vi "FPGA Read FIFO By Name - U32.vi"(6 "Timeout (ms)":u32=5000, 8 "error in (no error)":errorcluster, 9 "Number of Elements":u32, 10 "FIFO":string, 11 "FPGA Session In":refnum<class "FPGA Interface Base.lvclass">) -> (0 "error out":errorcluster, 1 "Elements Remaining":u32, 2 "Data":u32[](array[numeric]), 3 "FPGA Session Out":refnum<class "FPGA Interface Base.lvclass">)   [LabVIEW 2010, in "FPGA Interface Base.lvclass"]
doc: "Reads from a FIFO of unsigned 32-bit integers."
uses:
  <userlib>/_FPGA Interface Advanced Tools/FPGA Interface Base/FPGA Interface Base.lvclass
  <vilib>/rvi/DataTransferAndStorage/Container/Common/niFpgaDataTypeControl.ctl
  <userlib>/_FPGA Interface Advanced Tools/FPGA Interface Base/FPGA Interface Base.lvclass/FPGA Interface Base.ctl
  <vilib>/Utility/error.llb/Error Cluster From Error Code.vi
  <userlib>/_FPGA Interface Advanced Tools/FPGA Interface Base/Accessors/FPGA Read Session.vi
  <userlib>/_FPGA Interface Advanced Tools/FPGA Interface Wrapper/FPGA Interface Wrapper.lvlib
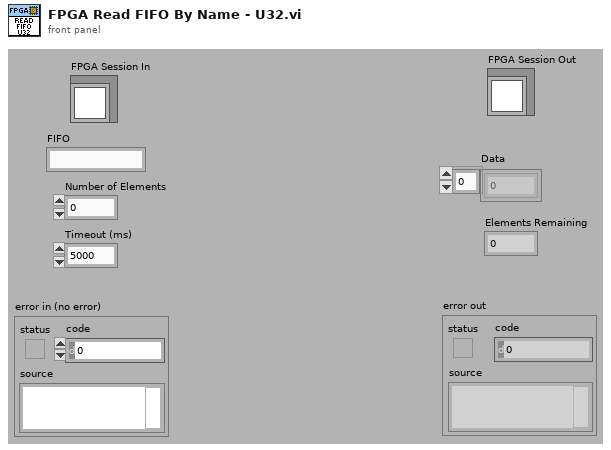
[diagram p1: front panel]
types:
  T1 = typedef "niFpgaDataTypeControl.ctl" = enum32{"Boolean", "I8", "I16", "I32", "I64", "U8", "U16", "U32", "U64", "FXP", "CustomControl"}
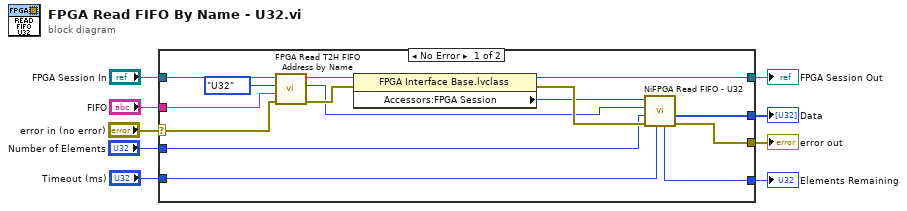
[diagram p0: block diagram]
diagram:
  n1 = case shown="No Error" "error in (no error)" {
    selector: "error in (no error)" -> [w17 w26]
    tunnel: [w20 w26] -> w2
    tunnel: [w21 w25] -> w4
    tunnel: [w24 _] -> w3
    tunnel: "FPGA Session In" -> [w19 w25]
    tunnel: "FIFO" -> [w16 _]
    tunnel: [w12 _] -> w1
    tunnel: "Number of Elements" -> [w11 _]
    tunnel: "Timeout (ms)" -> [w10 _]
    frame No Error {
      n2 = call <userlib>:"FPGA Read T2H FIFO Address by Name.vi"("error in (no error)"=w17, "Name"=w16, "Data Type"=niFpgaDataTypeControl."U32", "FPGA Interface Base in"=w19) -> ("error out"=w14:errorcluster, "Address"=w13:u32, "FPGA Interface Base out"=w18:refnum<class "FPGA Interface Base.lvclass">)  [unwired: 4 in, 1 out]
      n3 = property class="FPGA Interface Base.lvclass"(reference=w18, error in=w14) -> (reference out=w21:refnum<class "FPGA Interface Base.lvclass">, error out=w23:errorcluster, "Accessors:FPGA Session"=w22:u32)
      n4 = call <userlib>:"NiFPGA Read FIFO - U32.vi"("Timeout"=w10, "error in (no error)"=w23, "Number of Elements"=w11, "FIFO"=w13, "Session"=w22) -> ("error out"=w20:errorcluster, "Data"=w24:u32[], "Elements Remaining"=w12:u32)  [unwired: 3 in, 1 out]
    }
    frame Error {
    }
  }
  "error out" <- w2
  "FPGA Session Out" <- w4
  "Data" <- w3
  "Elements Remaining" <- w1
